vi "Test_extPicture.vi"() -> ()   [LabVIEW 2016]
uses:
  System.Windows.Forms
  USER32.DLL
panel:
  in  "PictureBox":refnum<k24>(container)
  out "*(type *) &x 2":u32
  out "Numeric":u32
  out "lpszWindowName":string
  out "hWnd 3":u32
  out "error out 2":errorcluster
  out "hWnd 2":u32
  out "hWnd":u32
  out "2D Picture":picture
  in  "Script":string
  in  "Media Source":string="rtsp://admin:admin@192.168.1.108/cam/realmonitor?channel=1&subtype=1"
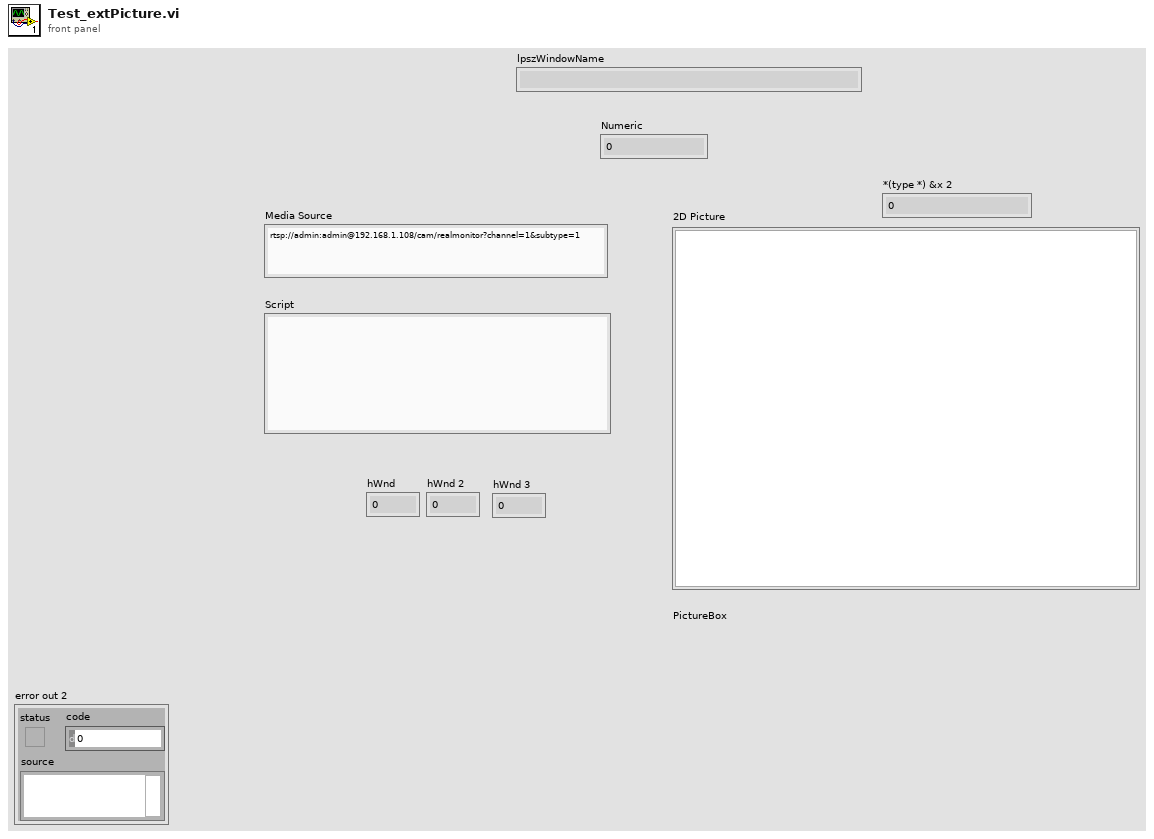
[diagram p1: front panel]
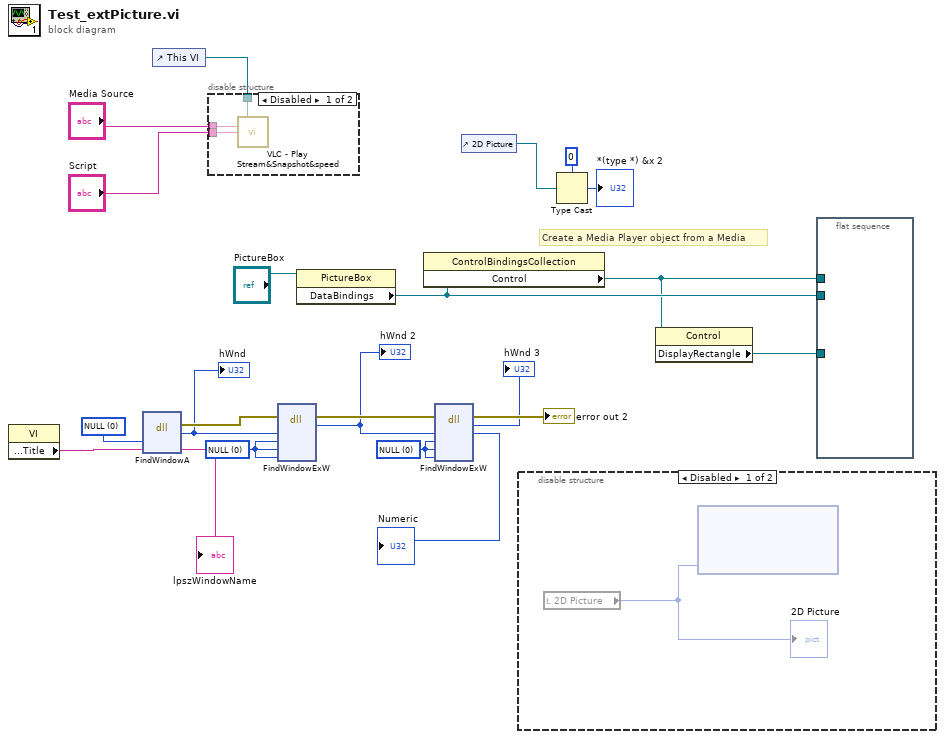
[diagram p0: block diagram]
diagram:
  w14 = 0 items=["NULL"]
  w18 = 0 items=["NULL"]
  w8 = 0 items=["NULL"]
  # "Create a Media Player object from a Media"
  n1 = property class="VI"() -> ("Front Panel Window:Title"=w19:string)  [unwired: 2 in, 2 out]
  n2 = dll-call lib="USER32.DLL" fn="FindWindowA" label="FindWindow"("lpszClassName"=w8, "lpszWindowName"=w19) -> (error out=w17:errorcluster, "hWnd"=w9:u32, "lpszWindowName"=→"lpszWindowName":string)  [unwired: 4 in, 1 out]
  "hWnd" <- w9
  n3 = control-ref of="This VI"() -> (w20:refnum<vi>)
  n4 = disable-structure shown="Disabled" {
    disable-tunnel: "Media Source" -> [w25 _]
    disable-tunnel: "Script" -> [w24 _]
    disable-tunnel: w20 -> [w23 _]
    frame Disabled {
      n5 = call "VLC - Play Stream&Snapshot&speed.vi"(1:w23, "Media Source"=w25, "Script"=w24) -> ()  [unwired: 12 in, 1 out]
    }
    frame Enabled {
    }
  }
  n6 = dll-call lib="user32.dll" fn="FindWindowExW" label="FindWindowEx"(error in=w17, "hwndParent"=w9, "hwndChildAfter"=w18, "lpszClassName"=w18, "lpszWindowName"=w18) -> (error out=w16:errorcluster, "hWnd"=w15:u32)  [unwired: 6 in, 1 out]
  "hWnd 2" <- w15
  n7 = property class="PictureBox"(reference="PictureBox") -> ("DataBindings"=w3:refnum<k24>)  [unwired: 1 in, 2 out]
  n8 = property class="ControlBindingsCollection"(reference=w3) -> ("Control"=w2:refnum<k24>)  [unwired: 1 in, 2 out]
  n9 = dll-call lib="user32.dll" fn="FindWindowExW" label="FindWindowEx"(error in=w16, "hwndParent"=w15, "hwndChildAfter"=w14, "lpszClassName"=w14, "lpszWindowName"=w14) -> (error out=→"error out 2":errorcluster, "hWnd"=→"hWnd 3":u32, "hwndParent"=→"Numeric":u32)  [unwired: 5 in, 1 out]
  n10 = control-ref of="2D Picture"() -> (w7:refnum<vi>)
  n11 = disable-structure shown="Disabled" {
    frame Disabled {
      n12 = local read "2D Picture"() -> (w26:picture)
      "2D Picture" <- w26
      n13 = node(w26) -> (w27:refnum<k24>)  [unwired: 3 in, 2 out]
    }
    frame Enabled {
    }
  }
  n14 = Type Cast(type=u32 0 ("hwndParent"), x=w7) -> (*(type *) &x=→"*(type *) &x 2":u32)
  n15 = property class="Control"(reference=w2) -> ("DisplayRectangle"=w1:refnum<k24>)  [unwired: 1 in, 2 out]
  n16 = flat-sequence {
    tunnel: w3 -> [_]
    tunnel: w2 -> [_]
    tunnel: w1 -> [_]
    frame #0 {
    }
  }
